vi "format_error_string.vi"(8 "error in (no error)":errorcluster) -> (0 "error out":errorcluster, 2 "error_string":string)   [LabVIEW 2021, in "system.logging.lvclass"]
uses:
  system.logging.lvclass
  system.logging.lvclass/system.logging.ctl
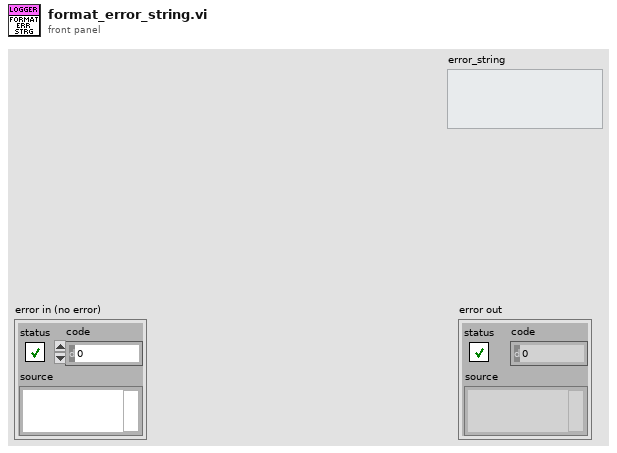
[diagram p1: front panel]
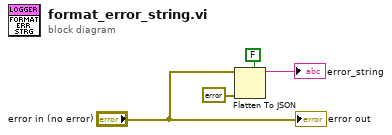
[diagram p0: block diagram]
diagram:
  n1 = Flatten To JSON(enable LabVIEW extensions? (T)=FALSE, anything="error in (no error)", error in (no error)=errorcluster {"status"=FALSE, "code"=0, "source"=""}) -> (JSON string=→"error_string":string)  [unwired: 1 out]
  "error out" <- "error in (no error)"
